vi "SwapFields.vi"(8 "error in (no error)":errorcluster, 11 "BME68x in":refnum<class "BME68x.lvclass">) -> (0 "error out":errorcluster, 3 "BME68x out":refnum<class "BME68x.lvclass">)   [LabVIEW 2022 SP3, in "BME68x.lvlib" / "BME68x.lvclass"]
uses:
  BME68x.lvclass
  BME68x.lvclass/BME68x.ctl
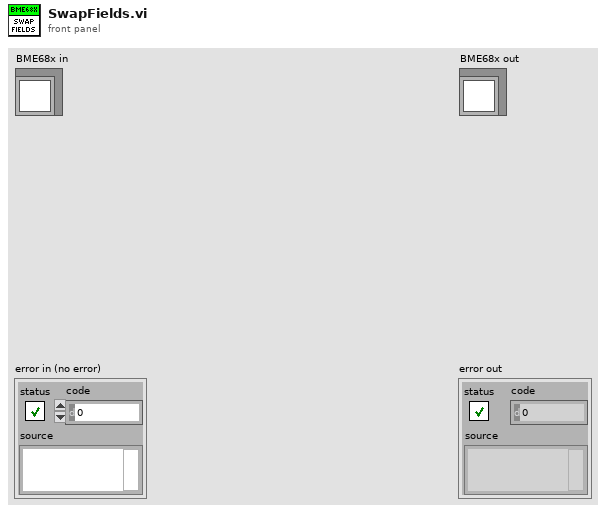
[diagram p1: front panel]
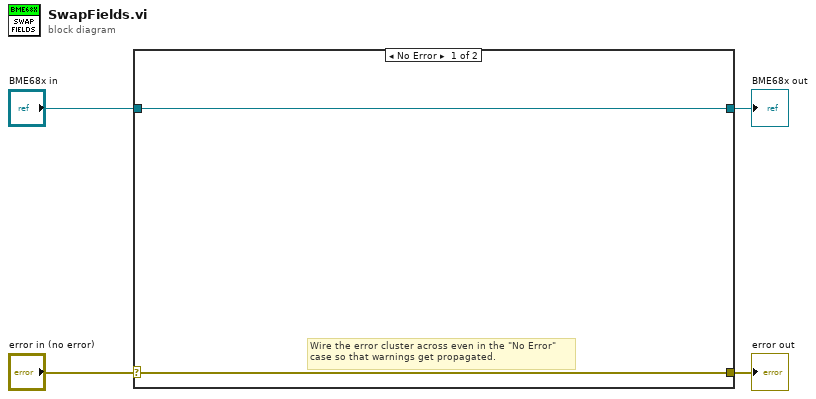
[diagram p0: block diagram]
diagram:
  n1 = case shown="No Error" "error in (no error)" {
    selector: "error in (no error)" -> [w5 w8]
    tunnel: [w5 w8] -> w3
    tunnel: [w6 w7] -> w1
    tunnel: "BME68x in" -> [w6 w7]
    frame No Error {
      # "Wire the error cluster across even in the \"No Error\"\ncase so that warnings get propagated."
    }
    frame Error {
    }
  }
  "error out" <- w3
  "BME68x out" <- w1
